vi "Add Message.vi"(8 "error in":errorcluster, 10 "New Msg":string, 11 "Sys Log in":refnum<class "System Log.lvclass">) -> (0 "error out":errorcluster, 3 "Sys Log out":refnum<class "System Log.lvclass">)   [LabVIEW 2016, in "System Log.lvclass"]
uses:
  System Log.lvclass
  System Log.lvclass/System Log.ctl
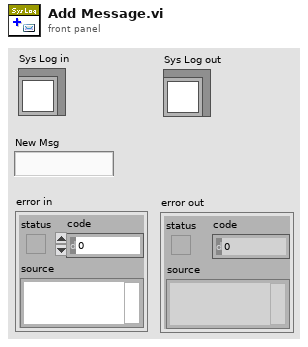
[diagram p1: front panel]
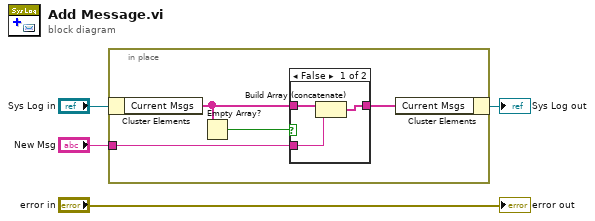
[diagram p0: block diagram]
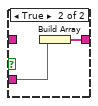
[diagram p2: hidden frame]
diagram:
  n1 = in-place {
    in-place-border: "New Msg" -> [w7]
    n2 = in-place-cluster #1("Sys Log in") -> ("Current Msgs"=w5:string[])
    n3 = Empty Array?(array=w5) -> (empty?=w8:bool)
    n4 = case shown="False" w8 {
      tunnel: w7 -> [w10 w13]
      tunnel: [w9 w12] -> w6
      tunnel: w5 -> [w11 _]
      frame False {
        n5 = Build Array (concatenate)(w11, w10) -> (w9:string[])
      }
      frame True {
        n6 = Build Array(w13) -> (w12:string[])
      }
    }
    n7 = in-place-cluster #1("Current Msgs"=w6) -> (→"Sys Log out":refnum<class "System Log.lvclass">)
  }
  "error out" <- "error in"
